vi "setLabel.vi"(8 "error in (no error)":errorcluster, 10 "label":string, 11 "Delay in":refnum<class "Delay.lvclass">) -> (0 "error out":errorcluster, 3 "Delay out":refnum<class "Delay.lvclass">)   [LabVIEW 2011, in "Tools.lvlib" / "Scripting.lvlib" / "Delay.lvclass"]
uses:
  Delay.lvclass
  Delay.lvclass/Delay.ctl
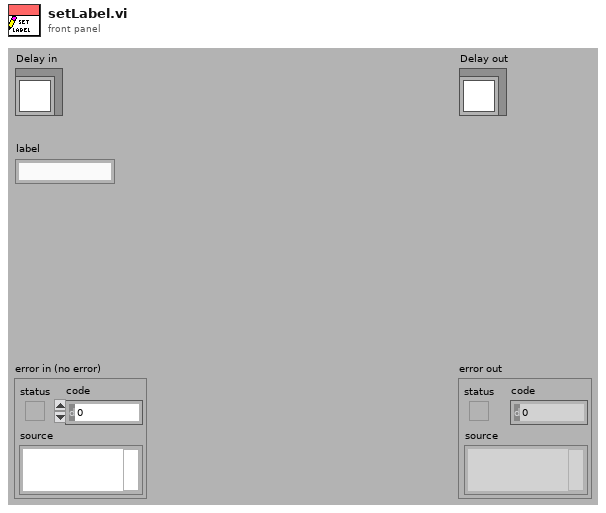
[diagram p1: front panel]
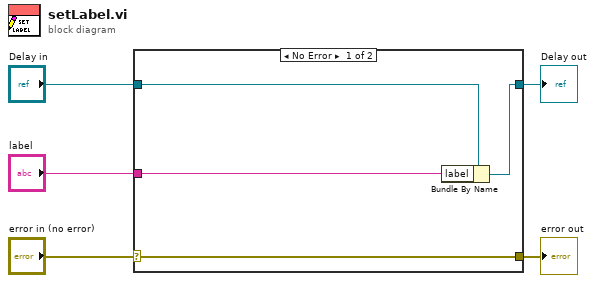
[diagram p0: block diagram]
diagram:
  n1 = case shown="No Error" "error in (no error)" {
    selector: "error in (no error)" -> [w9 w10]
    tunnel: [w9 w10] -> w4
    tunnel: [w7 w11] -> w2
    tunnel: "Delay in" -> [w8 w11]
    tunnel: "label" -> [w6 _]
    frame No Error {
      n2 = Bundle By Name(cluster=w8, "label"=w6) -> (w7:refnum<class "Delay.lvclass">)
    }
    frame Error {
    }
  }
  "error out" <- w4
  "Delay out" <- w2
